vi "Operate Directory.vi"(8 "error in (no error)":errorcluster, 9 "Directory Name":string, 10 "Directory Operation (0: Create Directory)":i32(ring) items=["Create Directory", "Change Directory", "Remove Directory"], 11 "VISA resource name":refnum<visa-resource-name>) -> (0 "error out":errorcluster, 3 "VISA resource name out":refnum<visa-resource-name>)   [LabVIEW 2012, in "Keysight B2980 Series.lvlib"]
doc: "Creates, changes or removes directory."
uses:
  Keysight B2980 Series.lvlib
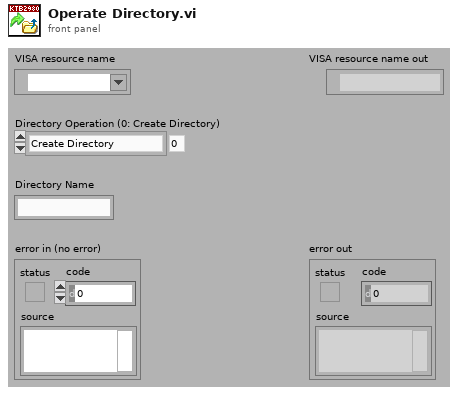
[diagram p1: front panel]
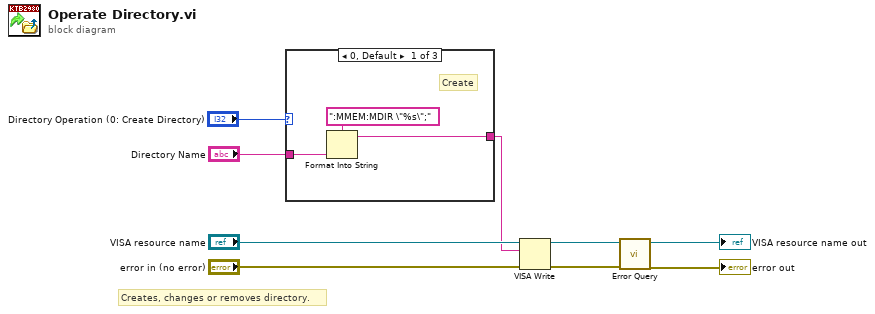
[diagram p0: block diagram]
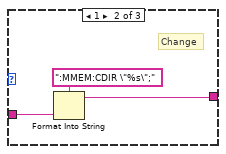
[diagram p2: hidden frame]
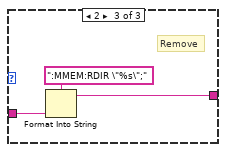
[diagram p3: hidden frame]
diagram:
  # "Creates, changes or removes directory."
  n1 = case shown="0, Default" "Directory Operation (0: Create Directory)" {
    tunnel: "Directory Name" -> [w11 w14 w17]
    tunnel: [w10 w13 w16] -> w1
    frame 0, Default {
      # "Create"
      n2 = Format Into String(format string=":MMEM:MDIR \"%s\";", w11) -> (resulting string=w10:string)  [unwired: 2 in, 1 out]
    }
    frame 1 {
      # "Change"
      n3 = Format Into String(format string=":MMEM:CDIR \"%s\";", w14) -> (resulting string=w13:string)  [unwired: 2 in, 1 out]
    }
    frame 2 {
      # "Remove"
      n4 = Format Into String(format string=":MMEM:RDIR \"%s\";", w17) -> (resulting string=w16:string)  [unwired: 2 in, 1 out]
    }
  }
  n5 = VISA Write(VISA resource name="VISA resource name", write buffer=w1, error in (no error)="error in (no error)") -> (VISA resource name out=w7:refnum<visa-resource-name>, error out=w6:errorcluster)  [unwired: 1 out]
  n6 = call "Error Query.vi"("error in (no error)"=w6, "VISA resource name"=w7) -> ("error out"=→"error out":errorcluster, "VISA resource name out"=→"VISA resource name out":refnum<visa-resource-name>)  [unwired: 8 out]
